vi "MotionProfiles_Control.vi"(8 "error in (no error)":errorcluster, 11 "MotionProfiles in":refnum<class "MotionProfiles.lvclass">) -> (0 "error out":errorcluster, 3 "MotionProfiles out":refnum<class "MotionProfiles.lvclass">)   [LabVIEW 2017, in "MotionProfiles.lvclass"]
uses:
  MotionProfiles.lvclass
  <vilib>/Rock Robotics/WPI/ThirdParty/Phoenix-LabVIEW/Motor Controller/Controls/CTRE_Phoenix_MotorControl_ControlMode.ctl
  MotionProfiles.lvclass/MotionProfiles.ctl
  MotionProfile_TalonSetValueEnum.ctl
  MotionProfile_InternalStateEnum.ctl
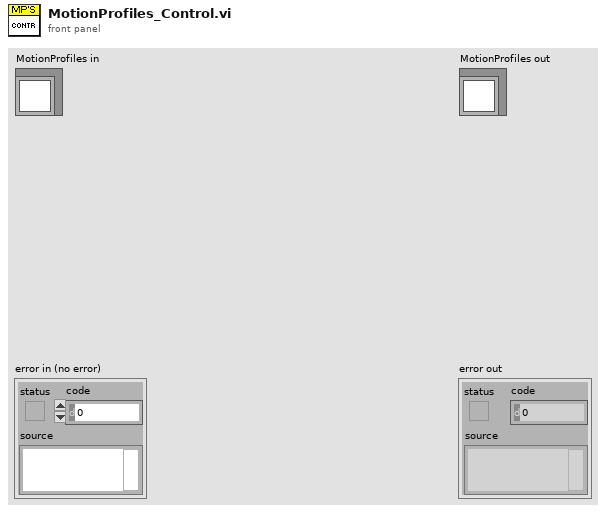
[diagram p1: front panel]
types:
  T1 = typedef "MotionProfiles.lvclass/MotionProfile_InternalStateEnum.ctl" = enum16{"Nothing", "Send Points to Talon", "Run Profile"}
  T2 = typedef "MotionProfiles.lvclass/MotionProfile_TalonSetValueEnum.ctl" = enum16{"Disable", "Enable", "Hold"}
  T3 = typedef "CTRE_Phoenix_MotorControl_ControlMode.ctl" = u16
  T4 = typedef "WPI_MotorControlDeviceRef.ctl" = cluster{"DeviceStatus":errorcluster, "Type":T5, "PWM":cluster{"PWM Channel":T6, "DeadBand":T7}, "CAN":cluster{"Device Number":u8, "SetOutput VI Ref":variant, "GetOutput VI Ref":variant, "Enable VI Ref":variant, "Disable VI Ref":variant, "Data":variant}, "Invert":bool, "DIO PWM":cluster{"PWM \"Enable\" Channel":T6, "DIOChannel":T8, "PWM Rate":dbl}}
  T5 = typedef "WPI_MotorControlType.ctl" = enum16{"PWM", "CAN", "DIO PWM"}
  T6 = typedef "FPGA_DIOPWMChannel.ctl" = enum8{"PWM 0", "PWM 1", "PWM 2", "PWM 3", "PWM 4", "PWM 5", "PWM 6", "PWM 7", "PWM 8", "PWM 9", "PWM MXP 0", "PWM MXP 1", "PWM MXP 2", "PWM MXP 3", "PWM MXP 4", "PWM MXP 5", "PWM MXP 6", "PWM MXP 7", "PWM MXP 8", "PWM MXP 9", "Invalid"}
  T7 = typedef "WPI_PWMDeadband.ctl" = cluster{"Name":string, "maxPositivePwm":i32, "minPositivePwm":i32, "centerPwm":i32, "maxNegativePwm":i32, "minNegativePwm":i32, "angularRange":u16}
  T8 = typedef "FPGA_DIOChannel.ctl" = enum8{"DIO 0", "DIO 1", "DIO 2", "DIO 3", "DIO 4", "DIO 5", "DIO 6", "DIO 7", "DIO 8", "DIO 9", "DIO MXP 0", "DIO MXP 1", "DIO MXP 2", "DIO MXP 3", "DIO MXP 4", "DIO MXP 5", "DIO MXP 6", "DIO MXP 7", "DIO MXP 8", "DIO MXP 9", "DIO MXP 10", "DIO MXP 11", "DIO MXP 12", "DIO MXP 13", "DIO MXP 14", "DIO MXP 15", "SPI Port CS1", "SPI Port CS2", "SPI Port CS3", "SPI Port MISO", "SPI Port MOSI", "Invalid"}
  T9 = cluster{"Top Buffer Remaining":i32, "Top Buffer Count":i32, "Bottom Buffer Count":i32, "Has Underrun?":bool, "Is Underrun?":bool, "Active Point Valid?":bool, "Is Last?":bool, "Profile Slot Select 0":i32, "Output Enable":i32, "Time Duration (ms)":i32, "Profile Slot Select 1":i32}
  T10 = typedef "MotionProfiles.lvclass/MotionProfile_TrajectoryPoint.ctl" = cluster{"Duration (ms)":u8, "Velocity (u/100ms)":dbl, "Position (units)":dbl, "Profile Slot Select":u8, "Is Last":bool, "Velocity Only":bool, "Zero Position":bool, "Compress Code":u8, "Same Velocity":i32, "Delta Position":i32, "Count":u8}
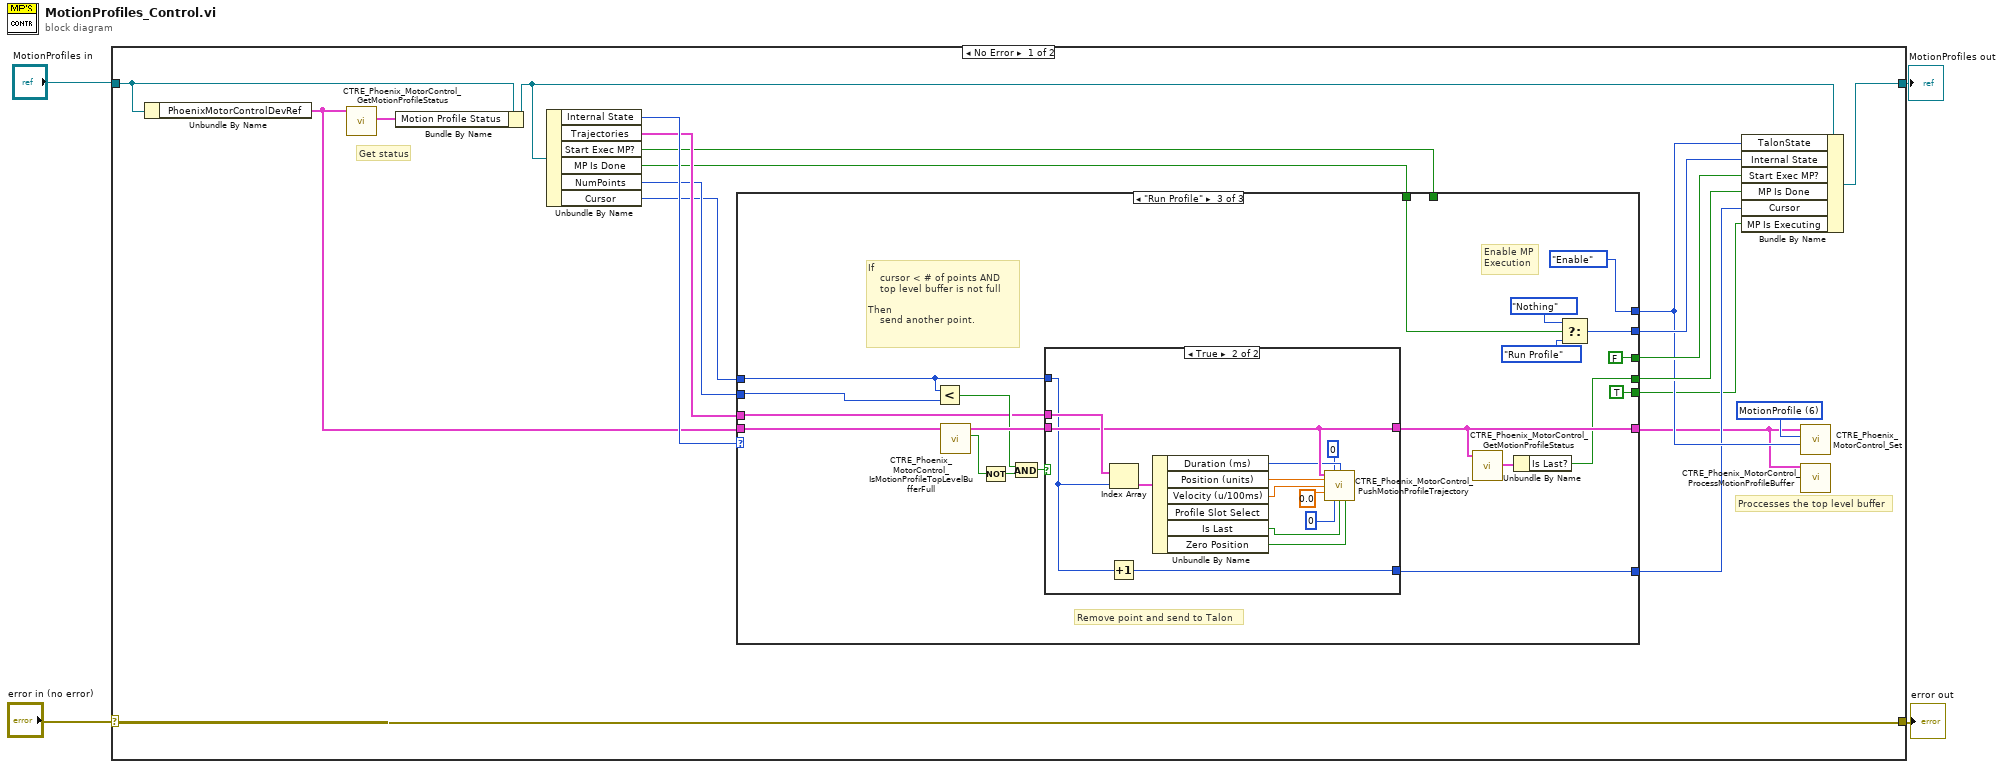
[diagram p0: block diagram]
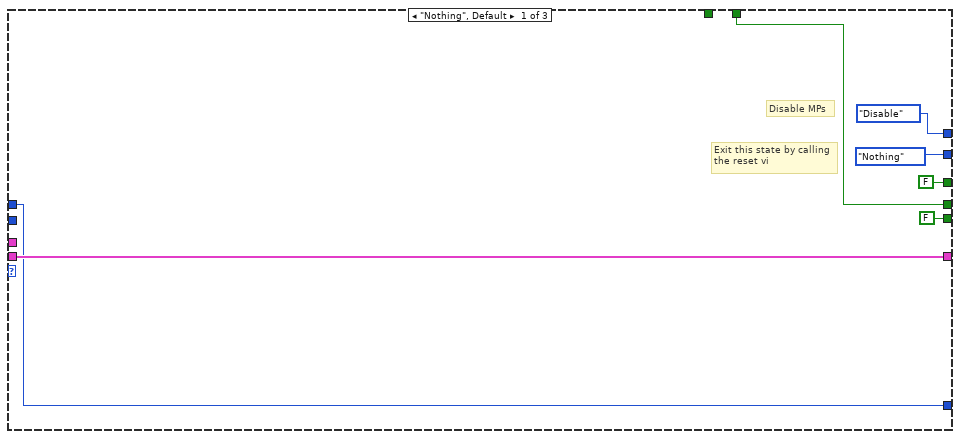
[diagram p2: hidden frame]
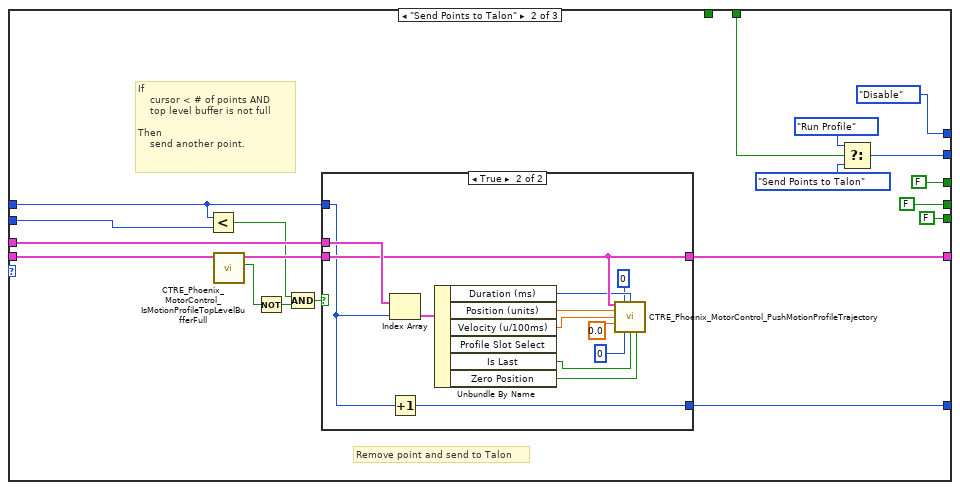
[diagram p3: hidden frame]
diagram:
  n1 = case shown="No Error" "error in (no error)" {
    selector: "error in (no error)" -> [w24 w102]
    tunnel: [w24 w102] -> w3
    tunnel: [w23 w101] -> w1
    tunnel: "MotionProfiles in" -> [w6 w101]
    frame No Error {
      w15 = T3 6 items=["PercentOutput"=0, "Position"=1, "Velocity"=2, "Current"=3, "Follower"=5, "MotionProfile"=6, "MotionMagic"=7, "MotionMagicArc"=8, "MotionProfileArc"=10, "Disabled"=15] ("Control Mode")
      # "Get status"
      # "Proccesses the top level buffer"
      n2 = Unbundle By Name(w6) -> ("PhoenixMotorControlDevRef"=w8:T4)
      n3 = call <vilib>:"CTRE_Phoenix_MotorControl_GetMotionProfileStatus.vi"("PhoenixMotorControlDevRef"=w8) -> ("Motion Profile Status"=w5:T9)  [unwired: 8 in, 2 out]
      n4 = Bundle By Name(cluster=w6, "Motion Profile Status"=w5) -> (w7:refnum<class "MotionProfiles.lvclass">)
      n5 = Unbundle By Name(w7) -> ("Internal State"=w22:T1, "Trajectories"=w21:T10[], "Start Exec MP?"=w20:bool, "MP Is Done"=w18:bool, "NumPoints"=w17:u32, "Cursor"=w11:u32)
      n6 = case shown="\"Run Profile\"" w22 {
        tunnel: [MotionProfile_InternalStateEnum."Nothing" ("Internal State") w48 w83] -> w14
        tunnel: [MotionProfile_TalonSetValueEnum."Disable" ("TalonSetValue") MotionProfile_TalonSetValueEnum."Disable" ("TalonSetValue") MotionProfile_TalonSetValueEnum."Enable" ("TalonSetValue")] -> w13
        tunnel: w21 -> [_ w47 w72]
        tunnel: w8 -> [w29 w39 w71]
        tunnel: w20 -> [w26 w42 _]
        tunnel: [FALSE ("Start Exec MP?") FALSE ("Start Exec MP?") FALSE] -> w19
        tunnel: w18 -> [_ _ w80]
        tunnel: w17 -> [_ w34 w73]
        tunnel: [w26 FALSE ("Mot Prof Active Is Last") w67] -> w16
        tunnel: [w29 w38 w69] -> w10
        tunnel: [w28 w36 w70] -> w12
        tunnel: w11 -> [w28 w35 w74]
        tunnel: [FALSE FALSE TRUE] -> w9
        frame "Nothing", Default {
          # "Exit this state by calling\nthe reset vi"
          # "Disable MPs"
        }
        frame "Send Points to Talon" {
          # "If \n    cursor < # of points AND\n    top level buffer is not full\n    \nThen \n    send another point."
          # "Remove point and send to Talon"
          n7 = Less?(x=w35, y=w34) -> (x < y?=w33:bool)
          n8 = call <vilib>:"CTRE_Phoenix_MotorControl_IsMotionProfileTopLevelBufferFull.vi"("PhoenixMotorControlDevRef"=w39) -> ("Is Motion Profile Top Level Buffer Full?"=w40:bool, "PhoenixMotorControlDevRef"=w37:T4)  [unwired: 8 in, 1 out]
          n9 = Not(x=w40) -> (.not. x?=w41:bool)
          n10 = Compound Arithmetic op=AND(w33, w41) -> (w43:bool)
          n11 = case shown="True" w43 {
            tunnel: w47 -> [_ w65]
            tunnel: [w52 w63] -> w38
            tunnel: w37 -> [w52 w63]
            tunnel: [w51 w54] -> w36
            tunnel: w35 -> [w51 w53]
            frame False {
            }
            frame True {
              n12 = Index Array(array=w65, index=w53) -> (element=w64:T10)
              n13 = Increment(x=w53) -> (x+1=w54:u32)
              n14 = Unbundle By Name(w64) -> ("Duration (ms)"=w62:u8, "Position (units)"=w60:dbl, "Velocity (u/100ms)"=w59:dbl, "Is Last"=w56:bool, "Zero Position"=w55:bool)  [unwired: 1 out]
              n15 = call <vilib>:"CTRE_Phoenix_MotorControl_PushMotionProfileTrajectory.vi"("PhoenixMotorControlDevRef"=w63, "profileSlotSelect1"=0, "durationMs"=w62, "position"=w60, "velocity"=w59, "headingDeg"=0.0, "profileSlotSelect0"=0, "isLastPoint?"=w56, "Zero Position?"=w55) -> ()  [unwired: 5 in, 2 out]
            }
          }
          n16 = Select(t=MotionProfile_InternalStateEnum."Run Profile" ("Internal State"), s=w42, f=MotionProfile_InternalStateEnum."Send Points to Talon" ("Internal State")) -> (s? t:f=w48:T1)
        }
        frame "Run Profile" {
          # "If \n    cursor < # of points AND\n    top level buffer is not full\n    \nThen \n    send another point."
          # "Remove point and send to Talon"
          # "Enable MP\nExecution"
          n17 = Less?(x=w74, y=w73) -> (x < y?=w75:bool)
          n18 = call <vilib>:"CTRE_Phoenix_MotorControl_IsMotionProfileTopLevelBufferFull.vi"("PhoenixMotorControlDevRef"=w71) -> ("Is Motion Profile Top Level Buffer Full?"=w77:bool, "PhoenixMotorControlDevRef"=w76:T4)  [unwired: 8 in, 1 out]
          n19 = Not(x=w77) -> (.not. x?=w78:bool)
          n20 = Compound Arithmetic op=AND(w75, w78) -> (w79:bool)
          n21 = case shown="True" w79 {
            tunnel: w72 -> [_ w100]
            tunnel: [w87 w98] -> w69
            tunnel: w76 -> [w87 w98]
            tunnel: [w86 w89] -> w70
            tunnel: w74 -> [w86 w88]
            frame False {
            }
            frame True {
              n22 = Index Array(array=w100, index=w88) -> (element=w99:T10)
              n23 = Increment(x=w88) -> (x+1=w89:u32)
              n24 = Unbundle By Name(w99) -> ("Duration (ms)"=w97:u8, "Position (units)"=w95:dbl, "Velocity (u/100ms)"=w94:dbl, "Is Last"=w91:bool, "Zero Position"=w90:bool)  [unwired: 1 out]
              n25 = call <vilib>:"CTRE_Phoenix_MotorControl_PushMotionProfileTrajectory.vi"("PhoenixMotorControlDevRef"=w98, "profileSlotSelect1"=0, "durationMs"=w97, "position"=w95, "velocity"=w94, "headingDeg"=0.0, "profileSlotSelect0"=0, "isLastPoint?"=w91, "Zero Position?"=w90) -> ()  [unwired: 5 in, 2 out]
            }
          }
          n26 = call <vilib>:"CTRE_Phoenix_MotorControl_GetMotionProfileStatus.vi"("PhoenixMotorControlDevRef"=w69) -> ("Motion Profile Status"=w68:T9)  [unwired: 8 in, 2 out]
          n27 = Unbundle By Name(w68) -> ("Is Last?"=w67:bool)
          n28 = Select(t=MotionProfile_InternalStateEnum."Nothing" ("Internal State"), s=w80, f=MotionProfile_InternalStateEnum."Run Profile" ("Internal State")) -> (s? t:f=w83:T1)
        }
      }
      n29 = Bundle By Name(cluster=w7, "TalonState"=w13, "Internal State"=w14, "Start Exec MP?"=w19, "MP Is Done"=w16, "Cursor"=w12, "MP Is Executing"=w9) -> (w23:refnum<class "MotionProfiles.lvclass">)
      n30 = call <vilib>:"CTRE_Phoenix_MotorControl_Set.vi"("Output"=w13, "Control Mode"=w15, "PhoenixMotorControlDevRef"=w10) -> ()  [unwired: 7 in, 2 out]
      n31 = call <vilib>:"CTRE_Phoenix_MotorControl_ProcessMotionProfileBuffer.vi"("PhoenixMotorControlDevRef"=w10) -> ()  [unwired: 13 in, 2 out]
    }
    frame Error {
    }
  }
  "error out" <- w3
  "MotionProfiles out" <- w1
